vi "TPNT_GetAll2Str.vi"() -> (2 "all":string)   [LabVIEW 2016]
uses:
  TPNT_CoreFunction.ctl
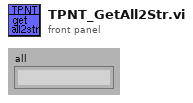
[diagram p1: front panel]
types:
  T1 = typedef "TPNT_CoreFunction.ctl" = enum16{"Reset", "Register", "Get Data", "Set Data", "Unregister", "Test", "Get Objects"}
  T2 = typedef "TPNT_Refnum.ctl" = refnum<vi>
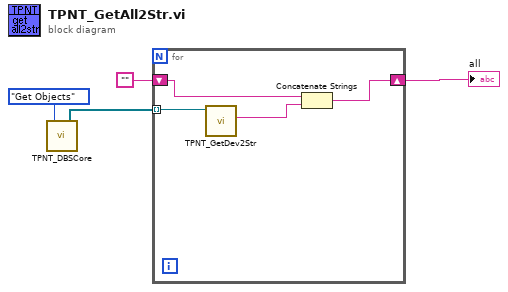
[diagram p0: block diagram]
diagram:
  n1 = call "TPNT_DBSCore.vi"("Function (Get Data)"=TPNT_CoreFunction."Get Objects") -> ("Objects"=w2:T2[])  [unwired: 4 in, 14 out]
  n2 = for {
    tunnel: w2 -> [w8] mode=indexing
    shift-right: [w6] -> w3
    shift-left: "" -> [w5]
    n3 = call "TPNT_GetDev2Str.vi"("Object Refnum In"=w8) -> ("str out"=w7:string)  [unwired: 1 in, 9 out]
    n4 = Concatenate Strings(w5, w7) -> (w6:string)
  }
  "all" <- w3
